vi "ec7.vi"() -> ()   [LabVIEW 2021]
uses:
  <vilib>/DAQmx/read.llb/DAQmx Read (Analog DBL 1Chan 1Samp).vi
  <vilib>/DAQmx/write.llb/DAQmx Write (Analog DBL 1Chan 1Samp).vi
  <vilib>/DAQmx/create/channels.llb/DAQmx Create Channel (AO-Voltage-Basic).vi
  <vilib>/DAQmx/create/channels.llb/DAQmx Create Channel (AI-Voltage-Basic).vi
  <vilib>/DAQmx/miscellaneous.llb/DAQmx Fill In Error Info.vi
  <vilib>/addons/control/pid/NI_PID_autopid.lvlib
panel:
  in  "File header":string="%Info. Blah. Blah.\n%Column 1: t [s]\n%Column 2: x [V]"
  in  "Data file name:":path=path "C:/temp/datafile_250816.lvm"
  in  "Start_stop_file_writing":bool
  in  "manual control":dbl
  in  "Stop":bool
  out "SP and PV":cluster{"initial PV":dbl, "SP1:":dbl}(graph)={"initial PV"=47.05872530934063, "SP1:"=47.05882352941177}
  in  "STime (s)":dbl=0.05 min=0.001 step=0.01 format="%#.3p"
  in  "PID Gains":T1={"proportional gain (Kc)"=15.221889907608013, "integral time (Ti, min)"=0.002027201803862475, "derivative time (Td, min)"=0.0002815558060920104} {"derivative time (Td, min)" format="%#.6g"; "integral time (Ti, min)" format="%#.6g"; "proportional gain (Kc)" format="%#.6g"}
  in  "SP:":dbl(slide)=47.05882352941177 min=0.0 max=0.0 scale=0.0..10.0
  in  "Autotune":bool
  in  "Accept Gain?":bool
  out "MV":dbl(graph)=18.823532635520305
  out "tuned PID gains":T1={"proportional gain (Kc)"=15.221889907608013, "integral time (Ti, min)"=0.002027201803862475, "derivative time (Td, min)"=0.0002815558060920104} {"derivative time (Td, min)" format="%#.6g"; "integral time (Ti, min)" format="%#.6g"; "proportional gain (Kc)" format="%#.6g"}
  in  "autotuning parameters":T2={"technique"=2, "controller type"=1, "control specification"=0, "amplitude"=1.0} {"amplitude" format="%.2f"; "control specification" items=["fast", "normal", "slow"]; "controller type" items=["P", "PI", "PID"]; "technique" items=["Step Open Loop", "Step Closed Loop", "Relay", "PID Relay"]}
  in  "Reinitialize":bool
  in  "setpoint\nweighting\n(beta)":dbl(knob)=3.8231445459877658 scale=0.0..1.0
  in  "Automatic":bool=TRUE
  in  "Set \nInitial Gain?":bool
  in  "Initial PID Gains":T1={"proportional gain (Kc)"=2.1923418207514507, "integral time (Ti, min)"=0.006000000284984708, "derivative time (Td, min)"=0.0} {"derivative time (Td, min)" format="%#.6g"; "integral time (Ti, min)" format="%#.6g"; "proportional gain (Kc)" format="%#.6g"}
  in  "setpoint\nweighting\n(gamma)":dbl(knob) scale=0.0..1.0
  out "tuning completed?":bool
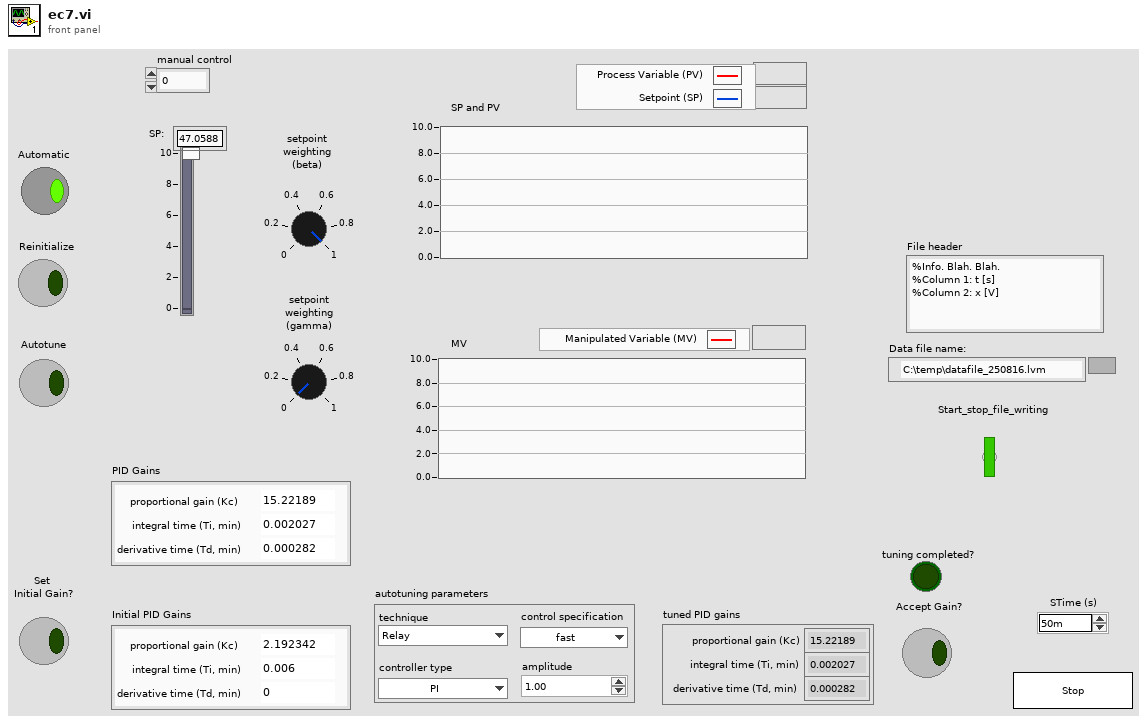
[diagram p1: front panel]
types:
  T1 = cluster{"proportional gain (Kc)":dbl, "integral time (Ti, min)":dbl, "derivative time (Td, min)":dbl}
  T2 = cluster{"technique":u16, "controller type":u16, "control specification":u16, "amplitude":dbl}
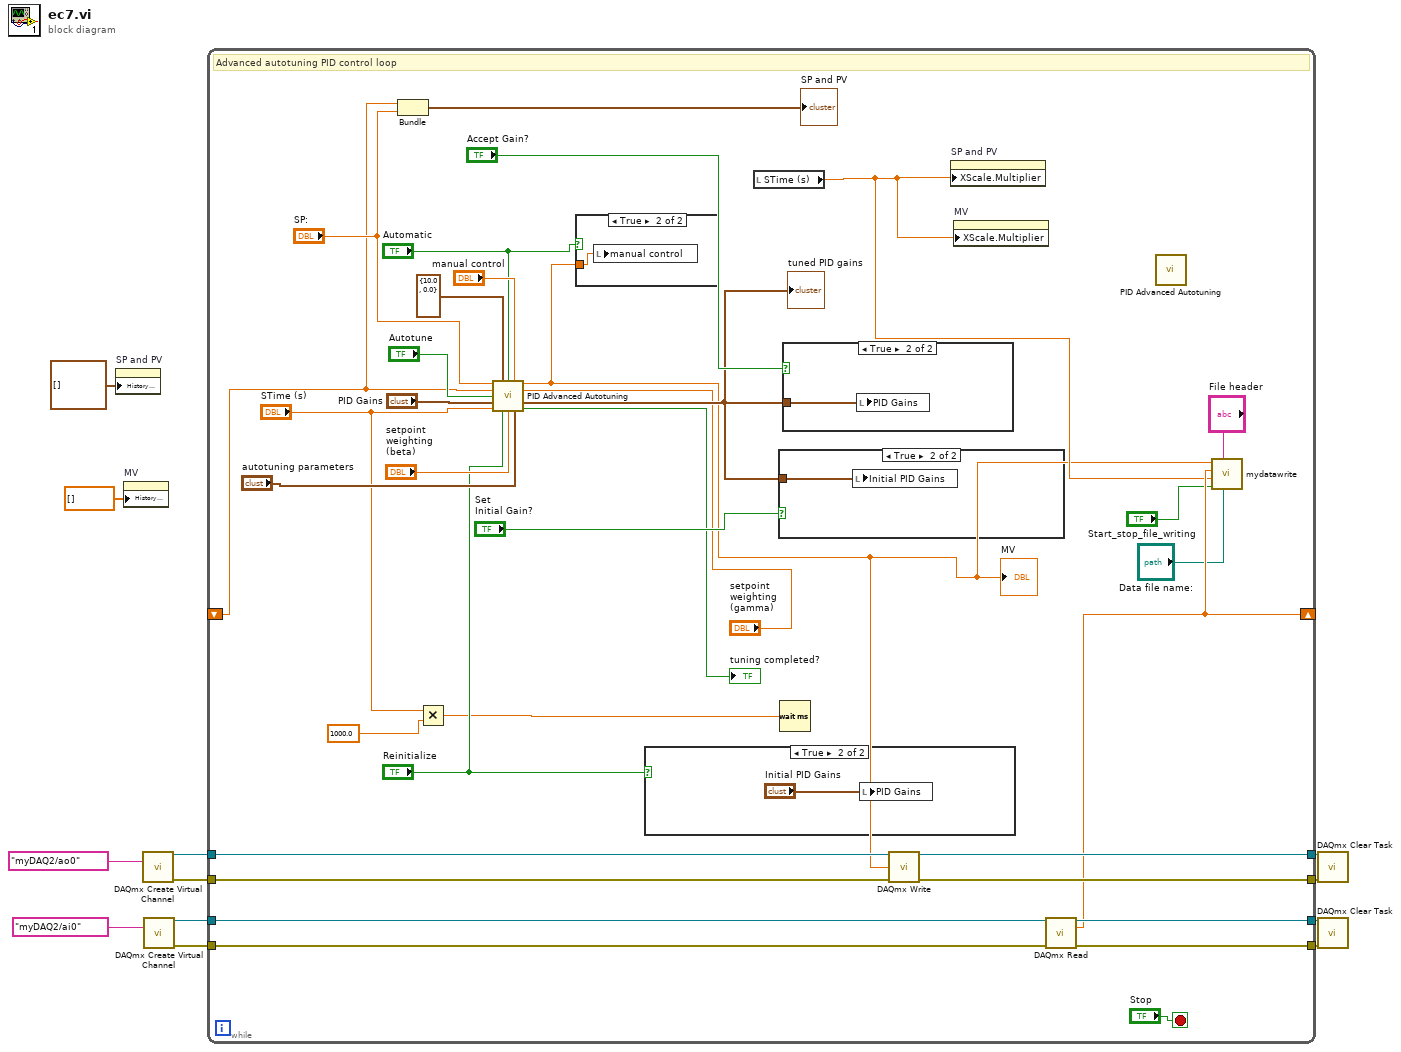
[diagram p0: block diagram]
diagram:
  n1 = property on="SP and PV" class="WFChart (strict)"("History Data"=cluster{"initial PV":dbl, "SP1:":dbl}[] []) -> ()  [unwired: 2 in, 2 out]
  n2 = property on="MV" class="WFChart (strict)"("History Data"=dbl[] []) -> ()  [unwired: 2 in, 2 out]
  n3 = call-poly <vilib>:"DAQmx Create Virtual Channel.vi"("physical channels"=tag "myDAQ2/ao0") -> ("task out"=w11:refnum<k21>, "error out"=w10:errorcluster)  [unwired: 13 in]
  n4 = call-poly <vilib>:"DAQmx Create Virtual Channel.vi"("physical channels"=tag "myDAQ2/ai0") -> ("task out"=w6:refnum<k21>, "error out"=w5:errorcluster)  [unwired: 13 in]
  n5 = while {
    tunnel: w11 -> [w32]
    tunnel: w10 -> [w31]
    tunnel: [w30] -> w9
    tunnel: [w29] -> w8
    tunnel: w6 -> [w28]
    tunnel: w5 -> [w27]
    tunnel: [w26] -> w4
    tunnel: [w25] -> w3
    shift-right: [w18] -> _
    shift-left: _ -> [w22]
    stop <- "Stop" stop-if-true
    # "Advanced autotuning PID control loop"
    n6 = Bundle("data"=w22, "SP:"="SP:") -> (→"SP and PV":cluster{"data":dbl, "SP:":dbl})  [unwired: 1 in]
    n7 = Multiply(x="STime (s)", y=1000.0 ("Simulation Time (times)")) -> (x*y=w37:dbl)
    n8 = call <vilib>:"PID Advanced Autotuning.vi"("setpoint"="SP:", "output range"=cluster{"output high":dbl, "output low":dbl} {"output high"=10.0, "output low"=0.0}, "auto? (F)"="Automatic", "manual control"="manual control", "process variable"=w22, "gamma"="setpoint\nweighting\n(gamma)", "autotune? (F)"="Autotune", "PID gains"="PID Gains", "dt (s)"="STime (s)", "reinitialize? (F)"="Reinitialize", "beta"="setpoint\nweighting\n(beta)", "autotuning parameters"="autotuning parameters") -> ("output"=w13:dbl, "tuned PID gains"=w34:T1, "tuning completed?"=→"tuning completed?":bool)  [unwired: 1 in]
    "MV" <- w13
    "tuned PID gains" <- w34
    n9 = case shown="True" "Automatic" {
      tunnel: w13 -> [_ w47]
      frame False {
      }
      frame True {
        n10 = local write "manual control"(w47) -> ()
      }
    }
    n11 = case shown="True" "Reinitialize" {
      frame False {
      }
      frame True {
        n12 = local write "PID Gains"("Initial PID Gains") -> ()
      }
    }
    n13 = local read "STime (s)"() -> (w17:dbl)
    n14 = case shown="True" "Set \nInitial Gain?" {
      tunnel: w34 -> [_ w49]
      frame False {
      }
      frame True {
        n15 = local write "Initial PID Gains"(w49) -> ()
      }
    }
    n16 = Wait (ms)(milliseconds to wait=w37) -> ()  [unwired: 1 out]
    n17 = case shown="True" "Accept Gain?" {
      tunnel: w34 -> [_ w50]
      frame False {
      }
      frame True {
        n18 = local write "PID Gains"(w50) -> ()
      }
    }
    n19 = call-poly <vilib>:"DAQmx Write.vi"("task/channels in"=w32, "data"=w13, "error in"=w31) -> ("task out"=w30:refnum<k21>, "error out"=w29:errorcluster)  [unwired: 10 in, 1 out]
    n20 = property on="SP and PV" class="WFChart (strict)"("XScale.Multiplier"=w17) -> ()  [unwired: 2 in, 2 out]
    n21 = property on="MV" class="WFChart (strict)"("XScale.Multiplier"=w17) -> ()  [unwired: 2 in, 2 out]
    n22 = call-poly <vilib>:"DAQmx Read.vi"("task/channels in"=w28, "error in"=w27) -> ("task out"=w26:refnum<k21>, "data"=w18:dbl, "error out"=w25:errorcluster)  [unwired: 11 in]
    n23 = call <vilib>:"PID Advanced Autotuning.vi"() -> ()  [unwired: 13 in, 3 out]
    n24 = call "mydatawrite.vi"("Data file name:"="Data file name:", "File header"="File header", "Start_stop_file_writing"="Start_stop_file_writing", "SampleTime"=w17, "Data2"=w18, "Data1"=w13) -> ()  [unwired: 6 in]
  }
  n25 = call <vilib>:"DAQmx Clear Task.vi"("task in"=w9, "error in"=w8) -> ()  [unwired: 13 in, 1 out]
  n26 = call <vilib>:"DAQmx Clear Task.vi"("task in"=w4, "error in"=w3) -> ()  [unwired: 13 in, 1 out]
